vi "Assign Point Ramping v1.3.vi"(4 "Accurus Ctrl Cluster":T1={"Stop Vacuum"=TRUE, "Vacuum Force"=0, "Max Limit [mmHg]"=600.0, "Slide in"=0, "Irrigation?"=TRUE} {"Slide in" scale=0.0..78.0; "Vacuum Force" min=0 max=78}, 5 "Ramp Time [sec]":dbl=3.0, 6 "L1 to L4 PID Cluster":T2={"L1 PID Gains"={"Kp"=0.005, "Kd"=0.5, "Ki"=0.0005}, "L2 PID Gains"={"Kp"=0.01, "Kd"=1.0, "Ki"=0.0005}, "L3 PID Gains"={"Kp"=0.05, "Kd"=1.0, "Ki"=0.0005}, "L4 PID Gains"={"Kp"=0.1, "Kd"=0.1, "Ki"=0.0005}}, 7 "Offset Home2RCM":dbl[](array[numeric])=[0.0, 0.0, 0.0, 0.0], 8 "Destination Posit Array [mm]":dbl[](array[numeric])=[0.0, 0.0, -3.0, 0.0], 9 "Previous Posit Array":dbl[](array[numeric])=[0.0, 0.0, 0.0, 0.0], 10 "error in":errorcluster, 11 "FPGA VI Reference In":refnum<k20>) -> (1 "Last L1 to L4 Posit":dbl[](array[numeric]), 2 "error out":errorcluster, 3 "FPGA VI Reference Out":refnum<k20>)   [LabVIEW 2010]
uses:
  <vilib>/Analysis/NI_AALBase.lvlib
  <vilib>/Analysis/1siggen.llb/Ramp Pattern by Samples.vi
  Subsystems/Global Variables.vi
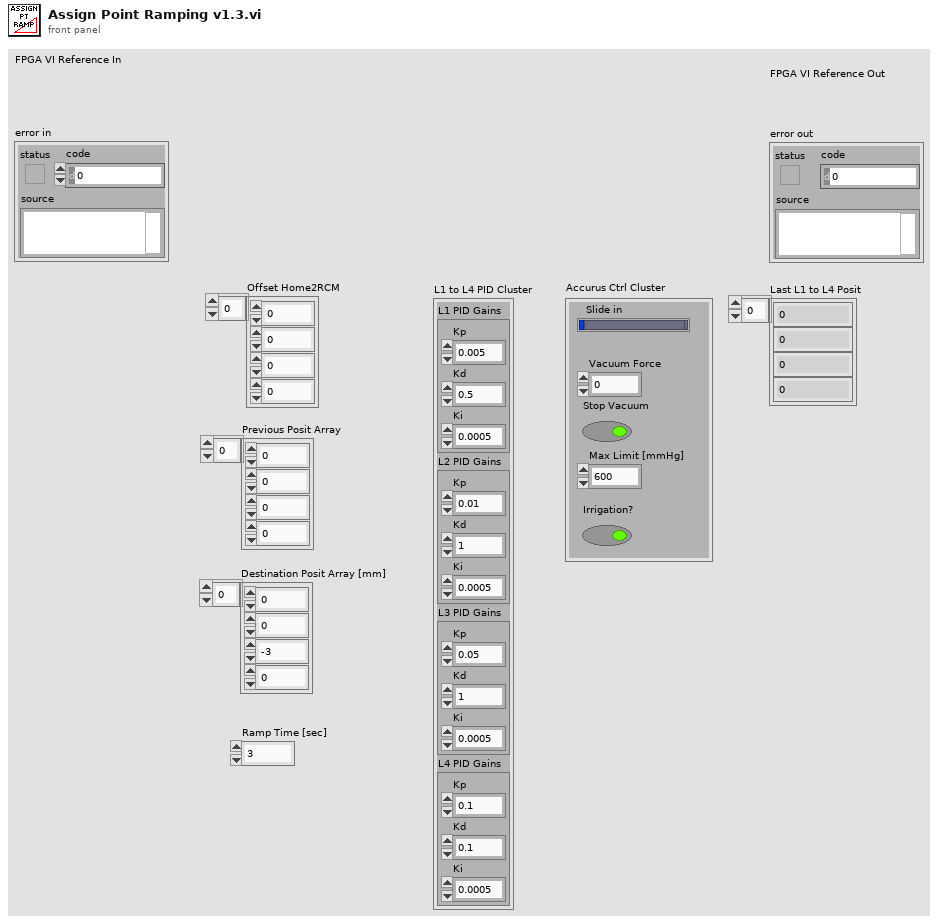
[diagram p1: front panel]
types:
  T1 = cluster{"Stop Vacuum":bool, "Vacuum Force":i8, "Max Limit [mmHg]":dbl, "Slide in":i8, "Irrigation?":bool}
  T2 = cluster{"L1 PID Gains":cluster{"Kp":dbl, "Kd":dbl, "Ki":dbl}, "L2 PID Gains":cluster{"Kp":dbl, "Kd":dbl, "Ki":dbl}, "L3 PID Gains":cluster{"Kp":dbl, "Kd":dbl, "Ki":dbl}, "L4 PID Gains":cluster{"Kp":dbl, "Kd":dbl, "Ki":dbl}}
  T3 = cluster{"Accurus button":bool[], "Accurus engaged?":bool, "Vacuum Force":i32, "Accurus Ch. A Vout":dbl, "Accurus Ch. B Vout":dbl, "Irrigation engaged?":bool}
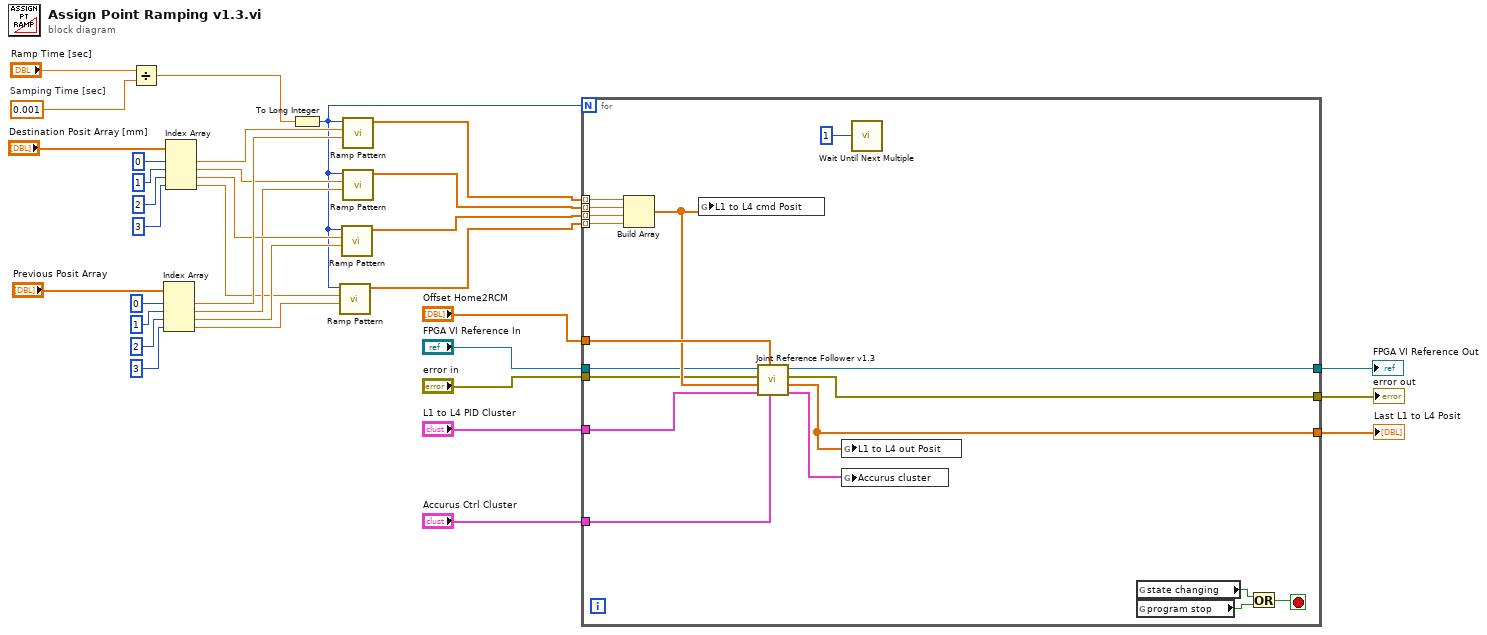
[diagram p0: block diagram]
diagram:
  w23 = 0.001  # Samping Time [sec]
  n1 = Divide(x="Ramp Time [sec]", y=w23) -> (x/y=w14:dbl)
  n2 = Index Array(array="Previous Posit Array", index #1=0 ("index"), index #2=1 ("index"), index #3=2 ("index"), index #4=3 ("index")) -> (element #1=w22:dbl, element #2=w18:dbl, element #3=w17:dbl, element #4=w16:dbl)
  n3 = Index Array(array="Destination Posit Array [mm]", index #1=0 ("index"), index #2=1 ("index"), index #3=2 ("index"), index #4=3 ("index")) -> (element #1=w21:dbl, element #2=w20:dbl, element #3=w19:dbl, element #4=w15:dbl)
  n4 = To Long Integer(number=w14) -> (32bit integer=w13:i32)
  n5 = call-poly <vilib>:"Ramp Pattern.vi"("start"=w16, "end"=w15, "samples"=w13) -> ("Ramp Pattern"=w9:dbl[])  [unwired: 7 in, 1 out]
  n6 = call-poly <vilib>:"Ramp Pattern.vi"("start"=w17, "end"=w19, "samples"=w13) -> ("Ramp Pattern"=w10:dbl[])  [unwired: 7 in, 1 out]
  n7 = call-poly <vilib>:"Ramp Pattern.vi"("start"=w22, "end"=w21, "samples"=w13) -> ("Ramp Pattern"=w12:dbl[])  [unwired: 7 in, 1 out]
  n8 = call-poly <vilib>:"Ramp Pattern.vi"("start"=w18, "end"=w20, "samples"=w13) -> ("Ramp Pattern"=w11:dbl[])  [unwired: 7 in, 1 out]
  n9 = for {
    N: w13 -> [_]
    tunnel: w12 -> [w52] mode=indexing
    tunnel: w11 -> [w51] mode=indexing
    tunnel: w10 -> [w50] mode=indexing
    tunnel: w9 -> [w49] mode=indexing
    tunnel: [w48] -> w1
    tunnel: [w47] -> w5
    tunnel: "Offset Home2RCM" -> [w46]
    tunnel: "L1 to L4 PID Cluster" -> [w45]
    tunnel: [w43] -> w7
    tunnel: "FPGA VI Reference In" -> [w35]
    tunnel: "error in" -> [w41]
    tunnel: "Accurus Ctrl Cluster" -> [w37]
    stop <- w38 stop-if-true
    n10 = Build Array(w52, w51, w50, w49) -> (w44:dbl[])
    n11 = global write "Global Variables.vi" "L1 to L4 cmd Posit"(w44) -> ()
    n12 = call "Joint Reference Follower v1.3.vi"("Accurus Ctrl Cluster"=w37, "Offset Home2RCM [deg/mm]"=w46, "PID Ctrl Cluster"=w45, "Ref Array [deg/mm]"=w44, "error in"=w41, "FPGA VI Reference In"=w35) -> ("Accurus Output Cluster"=w36:T3, "Output Posit Array [deg/mm]"=w43:dbl[], "error out"=w47:errorcluster, "FPGA VI Reference Out"=w48:refnum<k20>)  [unwired: 2 in]
    n13 = global write "Global Variables.vi" "L1 to L4 out Posit"(w43) -> ()
    n14 = global write "Global Variables.vi" "Accurus cluster"(w36) -> ()
    n15 = call "Wait Until Next Multiple"("Count(mSec)"=u32 1) -> ()  [unwired: 1 out]
    n16 = global read "Global Variables.vi" "state changing"() -> (w40:bool)
    n17 = global read "Global Variables.vi" "program stop"() -> (w39:bool)
    n18 = Or(x=w40, y=w39) -> (x .or. y?=w38:bool)
  }
  "error out" <- w5
  "Last L1 to L4 Posit" <- w7
  "FPGA VI Reference Out" <- w1
